vi "read.vi"(7 "LabVIEW Web Service Request":refnum<class "Web Request.lvclass">) -> (2 "slide":dbl)   [LabVIEW 2017]
uses:
  <vilib>/wsapi/Web Request.lvclass
  Globals.vi
panel:
  # "Use the Web Service Request input terminal to call the VIs on the Web Services palette. Do not remove it from the connector pane unless you don't need access to the palette."
  # "Each additional control wired to the connector pane will be available as an input in the URL. To include an indicator in terminal-mode output (the default setting), it must also be wired to the connector pane."
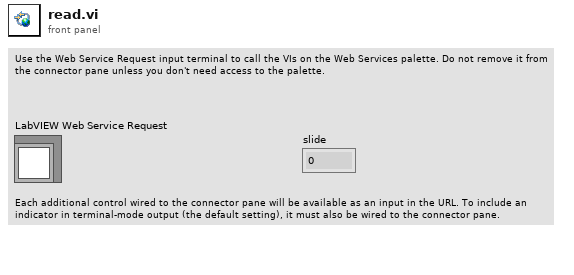
[diagram p1: front panel]
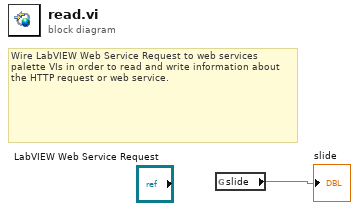
[diagram p0: block diagram]
diagram:
  # "Wire LabVIEW Web Service Request to web services palette VIs in order to read and write information about the HTTP request or web service."
  n1 = global read "Globals.vi" "slide"() -> (→"slide":dbl)
